vi "Determine Warnings-Edit2.vi"() -> ()   [LabVIEW 2014]
panel:
  in  "Max Wind Speed":dbl
  in  "Current Wind Speed":dbl
  out "Warning Text":string
  out "Warning?":bool
  out "Warning?":bool
  out "Warning Text":string
  in  "Min Temp":dbl
  in  "Max Temp":dbl
  in  "Current Temp":dbl
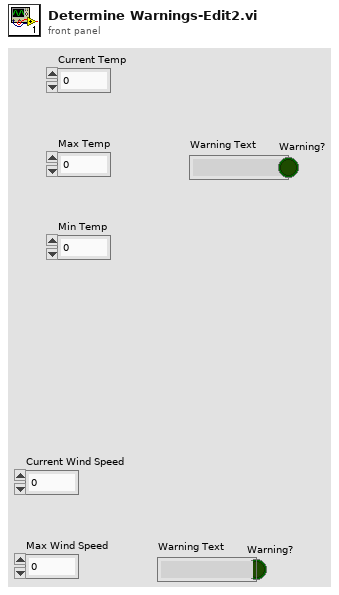
[diagram p1: front panel]
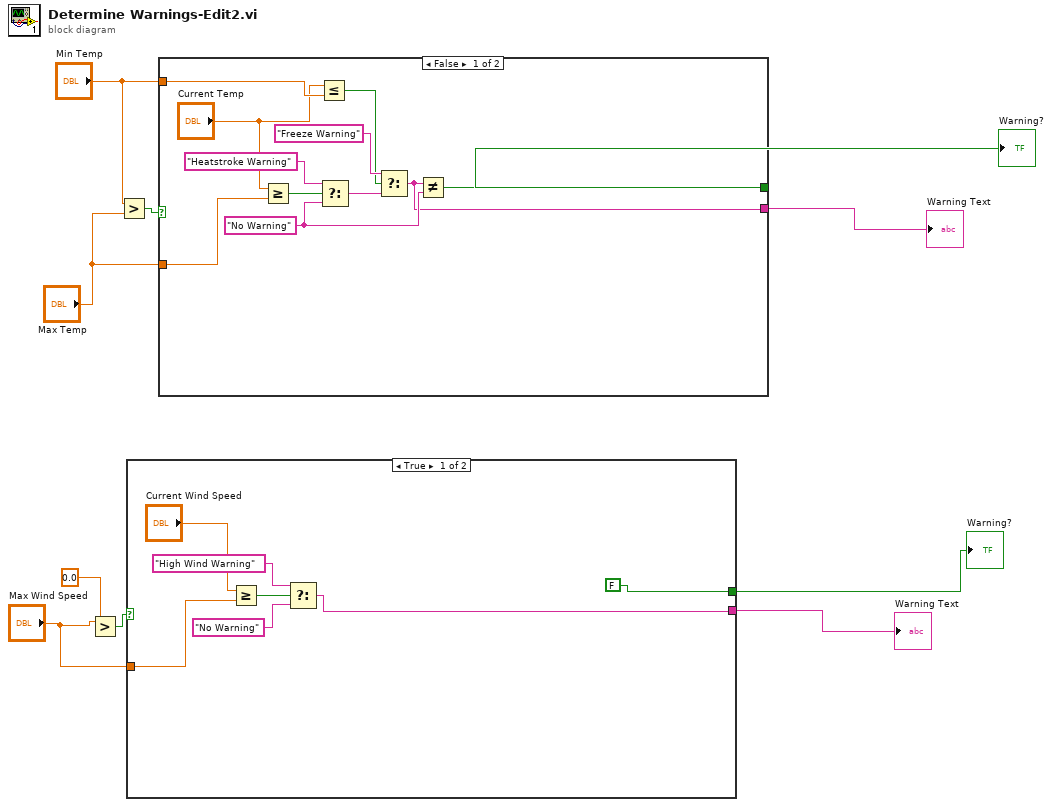
[diagram p0: block diagram]
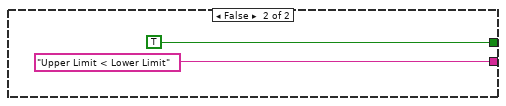
[diagram p2: hidden frame]
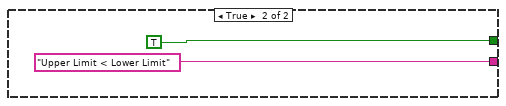
[diagram p3: hidden frame]
diagram:
  n1 = Greater?(x="Max Wind Speed", y=0.0) -> (0:w1:bool)
  n2 = Greater?(x="Min Temp", y="Max Temp") -> (0:w8:bool)
  n3 = case shown="True" w1 {
    tunnel: "Max Wind Speed" -> [w16 _]
    tunnel: [w12 "Upper Limit < Lower Limit"] -> w5
    tunnel: [FALSE TRUE] -> w4
    frame True {
      n4 = Greater Or Equal?(x="Current Wind Speed", y=w16) -> (x >= y?=w13:bool)
      n5 = Select(t="High Wind Warning", s=w13, f="No Warning") -> (s? t:f=w12:string)
    }
    frame False {
    }
  }
  "Warning Text" <- w5
  "Warning?" <- w4
  n6 = case shown="False" w8 {
    tunnel: "Min Temp" -> [w30 _]
    tunnel: "Max Temp" -> [w28 _]
    tunnel: [w21 TRUE] -> w7
    tunnel: [w20 "Upper Limit < Lower Limit"] -> w6
    frame False {
      w27 = "No Warning"
      n7 = Greater Or Equal?(x="Current Temp", y=w28) -> (x >= y?=w23:bool)
      n8 = Less Or Equal?(x="Current Temp", y=w30) -> (x <= y?=w22:bool)
      n9 = Select(t="Heatstroke Warning", s=w23, f=w27) -> (s? t:f=w26:string)
      n10 = Select(t="Freeze Warning", s=w22, f=w26) -> (s? t:f=w20:string)
      n11 = Not Equal?(x=w20, y=w27) -> (x != y?=w21:bool)
    }
    frame True {
    }
  }
  "Warning Text" <- w6
  "Warning?" <- w7
